vi "SetOccupancyParameters.vi"(8 "error in (no error)":errorcluster, 10 "Parameters":T1, 11 "OccupancyMap in":refnum<class "OccupancyMap.lvclass">) -> (0 "error out":errorcluster, 3 "OccupancyMap out":refnum<class "OccupancyMap.lvclass">)   [LabVIEW 2009, in "OccupancyMap.lvclass"]
uses:
  OccupancyMap.lvclass
  parameters.ctl
  OccupancyMap.lvclass/OccupancyMap.ctl
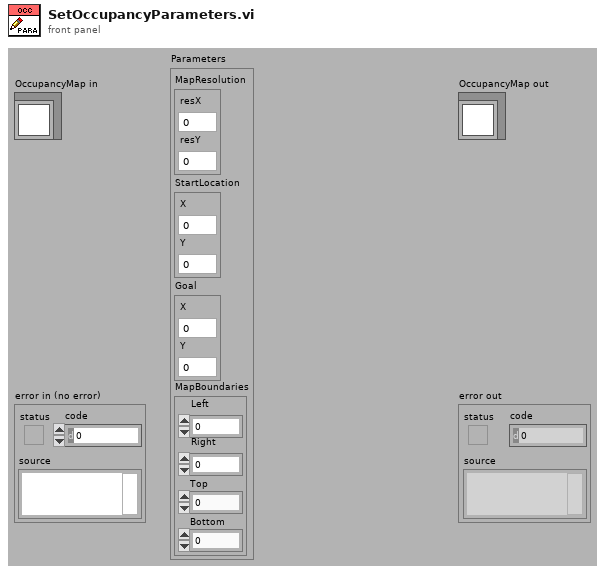
[diagram p1: front panel]
types:
  T1 = typedef "OccupancyMap.lvclass/parameters.ctl" = cluster{"MapResolution":cluster{"resX":dbl, "resY":dbl}, "StartLocation":cluster{"X":dbl, "Y":dbl}, "Goal":cluster{"X":dbl, "Y":dbl}, "MapBoundaries":cluster{"Left":dbl, "Right":dbl, "Top":dbl, "Bottom":dbl}}
  T2 = cluster{"Left":dbl, "Right":dbl, "Top":dbl, "Bottom":dbl}
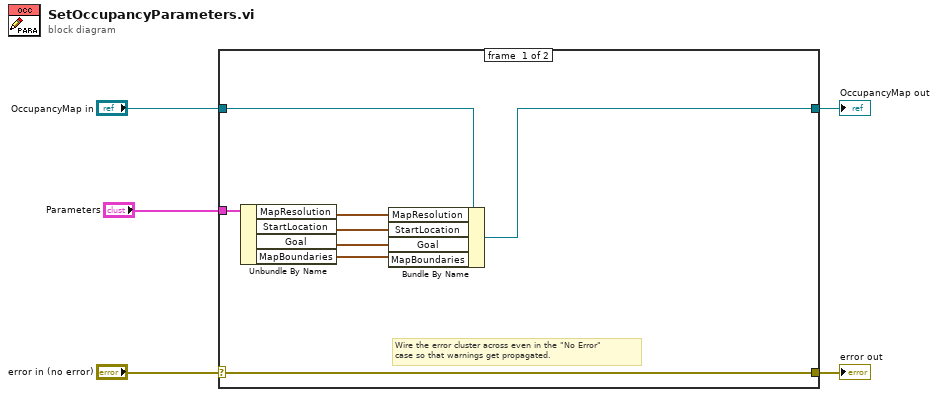
[diagram p0: block diagram]
diagram:
  n1 = case shown="No Error" "error in (no error)" {
    selector: "error in (no error)" -> [w13 w15]
    tunnel: [w13 w15] -> w4
    tunnel: [w6 w14] -> w2
    tunnel: "OccupancyMap in" -> [w7 w14]
    tunnel: "Parameters" -> [w12 _]
    frame #0 {
      # "Wire the error cluster across even in the \"No Error\"\ncase so that warnings get propagated."
      n2 = Unbundle By Name(w12) -> ("MapResolution"=w8:cluster{"resX":dbl, "resY":dbl}, "StartLocation"=w9:cluster{"X":dbl, "Y":dbl}, "Goal"=w10:cluster{"X":dbl, "Y":dbl}, "MapBoundaries"=w11:T2)
      n3 = Bundle By Name(cluster=w7, "MapResolution"=w8, "StartLocation"=w9, "Goal"=w10, "MapBoundaries"=w11) -> (w6:refnum<class "OccupancyMap.lvclass">)
    }
    frame #1 {
    }
  }
  "error out" <- w4
  "OccupancyMap out" <- w2
